vi "Receive Dashboard Packet.vi"(7 "connection ID out":refnum<k16>) -> ()   [LabVIEW 2014]
uses:
  Common Code/Dashboard Control Data.ctl
  Robot Global Data.vi
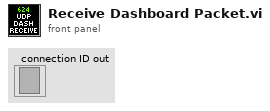
[diagram p1: front panel]
types:
  T1 = typedef "Dashboard Control Data.ctl" = cluster{"Boolean":bool}
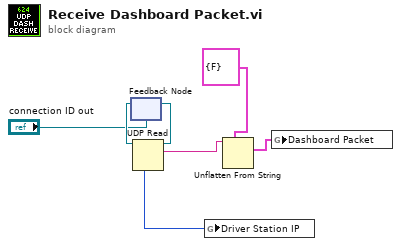
[diagram p0: block diagram]
diagram:
  n1 = feedback #1("connection ID out") -> (w6:refnum<k16>)
  n2 = UDP Read(connection ID=w6) -> (data out=w5:string, 3:w7:refnum<k16>, 6:w2:u32)  [unwired: 3 in, 2 out]
  n3 = feedback-in #1(w7) -> ()
  n4 = global write "Robot Global Data.vi" "Driver Station IP"(w2) -> ()
  n5 = Unflatten From String(type=T1 {"Boolean"=FALSE} ("DB Control Data"), binary string=w5) -> (value=w3:T1)  [unwired: 3 in, 2 out]
  n6 = global write "Robot Global Data.vi" "Dashboard Packet"(w3) -> ()
